vi "Read Supply Limits.vi"(8 "error in":errorcluster, 11 "6700 in":refnum<class "6700.lvclass">) -> (0 "error out":errorcluster, 3 "6700 out":refnum<class "6700.lvclass">)   [LabVIEW 2018, in "6700.lvlib" / "6700.lvclass"]
uses:
  6700.lvclass
  6700.lvclass/6700.ctl
  <instrlib>/Agilent N6700 Series/Agilent N6700 Series.lvlib
  builds/Power_Supply.lvlibp/Power Supply.lvclass
  C:/Users/Ron.Dexter.LUMINARTECH/Desktop/builds/Power_Supply.lvlibp/Power Supply.lvclass
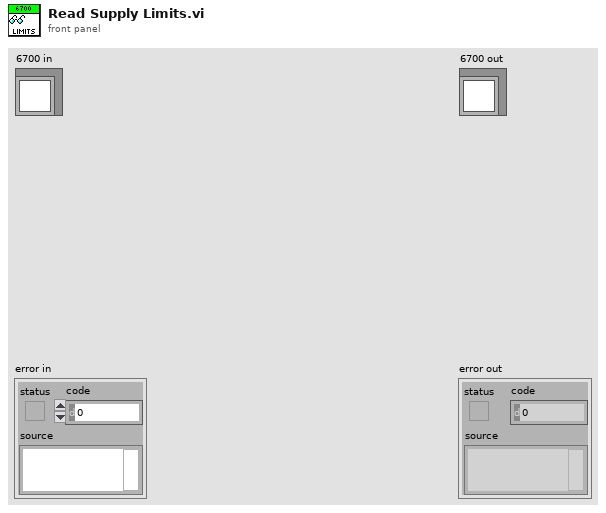
[diagram p1: front panel]
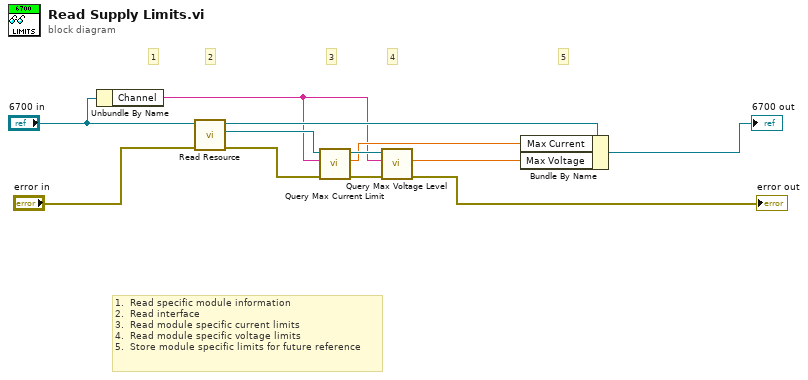
[diagram p0: block diagram]
diagram:
  # "1.  Read specific module information\n2.  Read interface\n3.  Read module specific current limits\n4.  Read module specific voltage limits\n5.  Store module specific limits for future reference"
  # "5"
  # "4"
  # "3"
  # "2"
  # "1"
  n1 = Unbundle By Name("6700 in") -> ("Channel"=w1:string)
  n2 = call "Read Resource.vi"("error in"="error in", "Power Supply in"="6700 in") -> ("error out"=w10:errorcluster, "Resource"=w6:refnum<visa-resource-name>, "Power Supply out"=w12:refnum<class "6700.lvclass">)  [unwired: 7 in]
  n3 = call <instrlib>:"Query Max Current Limit.vi"("error in (no error)"=w10, "Channel Name (1)"=w1, "VISA resource name"=w6) -> ("error out"=w9:errorcluster, "Max Current Limit"=w5:dbl, "VISA resource name out"=w7:refnum<visa-resource-name>)  [unwired: 6 in]
  n4 = call <instrlib>:"Query Max Voltage Level.vi"("error in (no error)"=w9, "Channel Name (1)"=w1, "VISA resource name"=w7) -> ("error out"=→"error out":errorcluster, "Max Voltage Level"=w4:dbl)  [unwired: 6 in, 1 out]
  n5 = Bundle By Name(cluster=w12, "Max Current"=w5, "Max Voltage"=w4) -> (→"6700 out":refnum<class "6700.lvclass">)
